vi "LUT_DropSpeedCurve.vi"() -> (0 "Init Data Out":fxp<+,10,10>[](array[numeric])=[1000.0, 910.0, 835.0, 772.0, 717.0, 670.0, 629.0, 593.0, 560.0, 532.0, 506.0, 482.0, 461.0, 441.0, 423.0, 407.0, 391.0, 377.0, 364.0, 352.0, 341.0, 330.0, 320.0, 311.0, 302.0, 294.0, 286.0, 278.0, 271.0, 265.0, 258.0, 252.0, 247.0, 241.0, 236.0, 231.0, 226.0, 222.0, 217.0, 213.0, 209.0, 205.0, 201.0, 198.0, 194.0, 191.0, 188.0, 185.0, 182.0, 179.0, 176.0, 173.0, 171.0, 168.0, 166.0, 163.0, 161.0, 159.0, 157.0, 154.0, 152.0, 150.0, 148.0, 147.0, 145.0, 143.0, 141.0, 140.0, 138.0, 136.0, 135.0, 133.0, 132.0, 130.0, 129.0, 127.0, 126.0, 125.0, 123.0, 122.0, 121.0, 120.0, 119.0, 117.0, 116.0, 115.0, 114.0, 113.0, 112.0, 111.0, 110.0, 109.0, 108.0, 107.0, 106.0, 105.0, 104.0, 104.0, 103.0, 102.0])   [LabVIEW 2018]
panel:
  in  "D":i32=20
  in  "C":i32=2
  in  "B":i32=18000
  in  "A":i32=2
  out "Graph":u16[](graph)=[1000, 910, 835, 772, 717, 670, 629, 593, 560, 532, 506, 482, 461, 441, 423, 407, 391, 377, 364, 352, 341, 330, 320, 311, 302, 294, 286, 278, 271, 265, 258, 252, 247, 241, 236, 231, 226, 222, 217, 213, 209, 205, 201, 198, 194, 191, 188, 185, 182, 179, 176, 173, 171, 168, 166, 163, 161, 159, 157, 154, 152, 150, 148, 147, 145, 143, 141, 140, 138, 136, 135, 133, 132, 130, 129, 127, 126, 125, 123, 122, 121, 120, 119, 117, 116, 115, 114, 113, 112, 111, 110, 109, 108, 107, 106, 105, 104, 104, 103, 102]
  # "For Initialization VI requirements and help, please read directions located on Block Diagram."
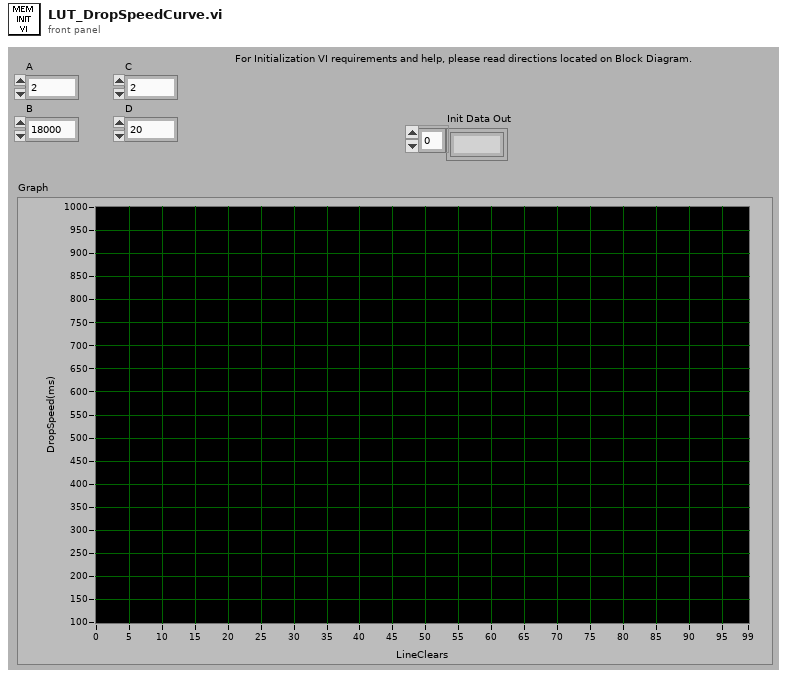
[diagram p1: front panel]
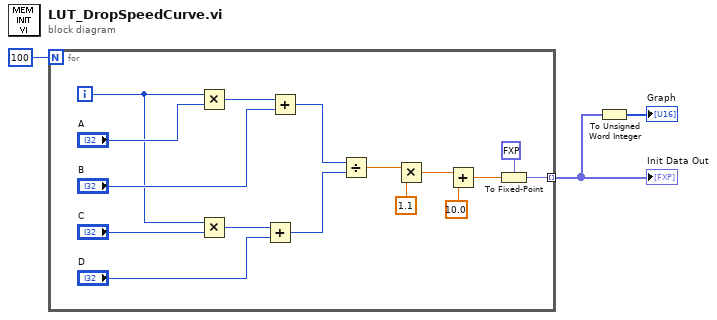
[diagram p0: block diagram]
diagram:
  n1 = for {
    N: 100 -> [_]
    tunnel: [w18] -> w2 mode=indexing
    i -> [w13]
    n2 = Multiply(x=w13, y="A") -> (x*y=w15:i32)
    n3 = Multiply(x=w13, y="C") -> (x*y=w11:i32)
    n4 = Add(x=w11, y="D") -> (x+y=w8:i32)
    n5 = Add(x=w15, y="B") -> (x+y=w9:i32)
    n6 = Divide(x=w9, y=w8) -> (x/y=w7:dbl)
    n7 = Multiply(x=w7, y=1.1) -> (x*y=w17:dbl)
    n8 = Add(x=w17, y=10.0) -> (x+y=w5:dbl)
    n9 = To Fixed-Point(fixed-point type=fxp<+,10,10> 0.0, number=w5) -> (fixed-point=w18:fxp<+,10,10>)
  }
  "Init Data Out" <- w2
  n10 = To Unsigned Word Integer(number=w2) -> (unsigned 16bit integer=→"Graph":u16[])
